vi "Initialize Inline Execution Units.vi"(8 "error in":errorcluster, 11 "RTStateVariables in":T1 {"Inline Execution Units"."Outgoing Data References"."Data Reference" format="%.0x"; "Inline Execution Units"."Incoming Data References" format="%.0x"}) -> (0 "error out":errorcluster, 3 "RTStateVariables out":T1 {"Inline Execution Units"."Outgoing Data References"."Data Reference" format="%.0x"; "Inline Execution Units"."Incoming Data References" format="%.0x"})   [LabVIEW 2023, in "Ballard MIL-STD-1553 Engine Support.lvlib" / "Custom Device.lvlib"]
uses:
  Custom Device.lvlib
  RTStateVariables.ctl
  <vilib>/NI/NIVS Inline Async API/_VS Inline Async API/VS Inline Async API/VS Inline Async API.lvclass
  Interfaces/Shared Resources/Shared Resources.lvclass
  Inline Execution Unit Runtime Information.ctl
  Interfaces/Execution Unit/Execution Unit.lvclass
  <vilib>/NI VeriStand/Custom Device API/Data Reference.ctl
  <vilib>/NI VeriStand/Custom Device API/Block Data Reference.ctl
  Asynchronous Execution Unit Runtime Information.ctl
  <vilib>/NI VeriStand/Custom Device Tools/Custom Device Utility Library/Custom Device Utility Library.lvlib
  <vilib>/NI VeriStand/Custom Device API/Custom Device API.lvlib
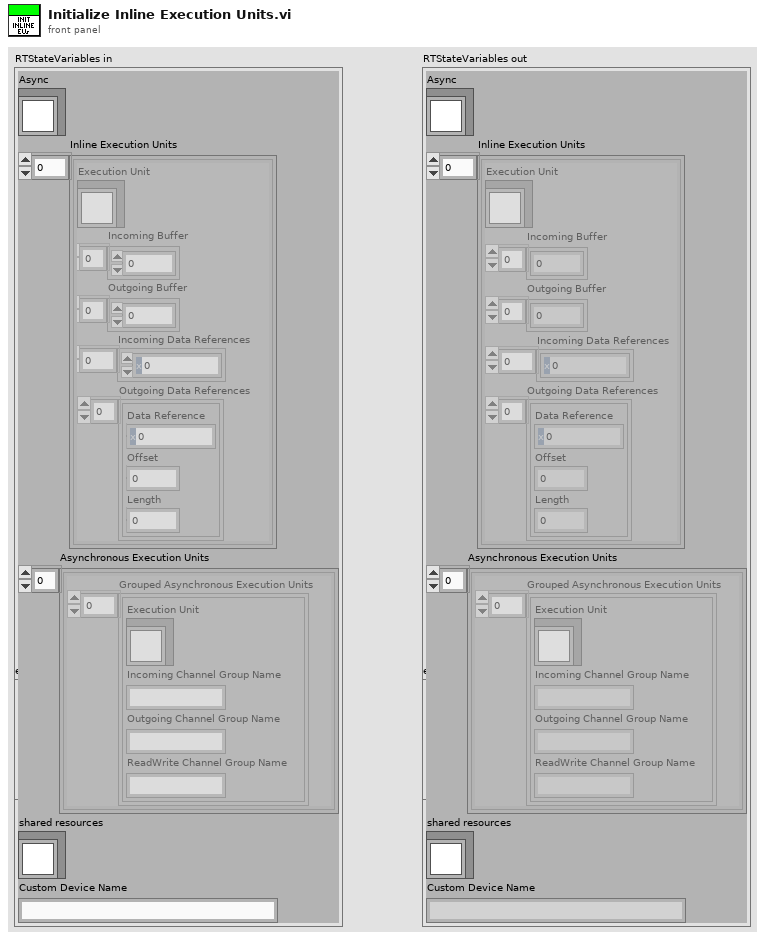
[diagram p1: front panel]
types:
  T1 = typedef "Ballard MIL-STD-1553 Engine Support.lvlib/Custom Device.lvlib/RTStateVariables.ctl" = cluster{"Async":refnum<class "VS Inline Async API.lvclass">, "Inline Execution Units":T2[], "Asynchronous Execution Units":cluster{"Grouped Asynchronous Execution Units":T5[]}[], "shared resources":refnum<class "Shared Resources.lvclass">, "Custom Device Name":string}
  T2 = typedef "Ballard MIL-STD-1553 Engine Support.lvlib/Custom Device.lvlib/Inline Execution Unit Runtime Information.ctl" = cluster{"Execution Unit":refnum<class "Execution Unit.lvclass">, "Incoming Buffer":dbl[], "Outgoing Buffer":dbl[], "Incoming Data References":T3[], "Outgoing Data References":T4[]}
  T3 = typedef "Custom Device API.lvlib/Data Reference.ctl" = i32
  T4 = typedef "Custom Device API.lvlib/Block Data Reference.ctl" = cluster{"Data Reference":T3, "Offset":u64, "Length":u64}
  T5 = typedef "Ballard MIL-STD-1553 Engine Support.lvlib/Custom Device.lvlib/Asynchronous Execution Unit Runtime Information.ctl" = cluster{"Execution Unit":refnum<class "Execution Unit.lvclass">, "Incoming Channel Group Name":string, "Outgoing Channel Group Name":string, "ReadWrite Channel Group Name":string}
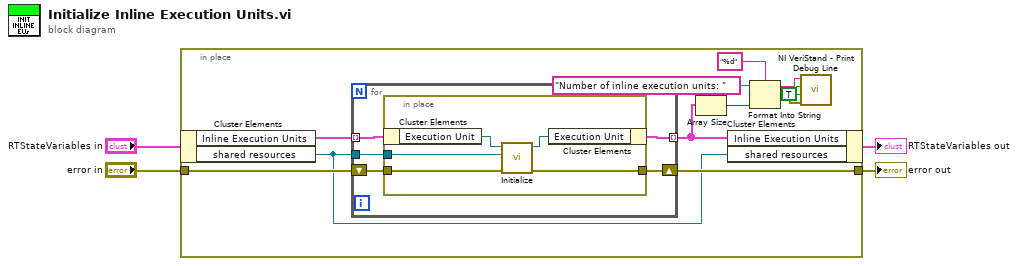
[diagram p0: block diagram]
diagram:
  n1 = in-place {
    in-place-border: "error in" -> [w14]
    in-place-border: [w13] -> w4
    w5 = TRUE ("Append newline? (T)")
    n2 = in-place-cluster #1("RTStateVariables in") -> ("Inline Execution Units"=w15:T2[], "shared resources"=w12:refnum<class "Shared Resources.lvclass">)
    n3 = for {
      tunnel: w15 -> [w18] mode=indexing
      tunnel: [w17] -> w8 mode=indexing
      shift-right: [w19] -> w13
      shift-left: w14 -> [w20]
      tunnel: w12 -> [w16]
      n4 = in-place {
        in-place-border: w20 -> [w25]
        in-place-border: [w24] -> w19
        in-place-border: w16 -> [w21]
        n5 = in-place-cluster #2(w18) -> ("Execution Unit"=w22:refnum<class "Execution Unit.lvclass">)
        n6 = call-dynamic "Initialize.vi"("error in (no error)"=w25, "shared resources"=w21, "Execution Unit in"=w22) -> ("error out"=w24:errorcluster, "Execution Unit out"=w23:refnum<class "Execution Unit.lvclass">)  [unwired: 7 in]
        n7 = in-place-cluster #2("Execution Unit"=w23) -> (w17:T2)
      }
    }
    n8 = Array Size(array=w8) -> (size(s)=w10:i32)
    n9 = in-place-cluster #1("Inline Execution Units"=w8, "shared resources"=w12) -> (→"RTStateVariables out":T1)
    n10 = Format Into String(format string="%d", initial string="Number of inline execution units: ", w10) -> (resulting string=w6:string, error out=w11:errorcluster)  [unwired: 1 in]
    n11 = call <vilib>:"NI VeriStand - Print Debug Line.vi"("error in (no error)"=w11, "Append newline? (T)"=w5, "Add to log file? (F)"=w5, "Message"=w6) -> ()  [unwired: 7 in, 1 out]
  }
  "error out" <- w4
